vi "EQR reanalysis.vi"() -> ()   [LabVIEW 2015, in "VIPM2.lvlib"]
doc: "El reanàlisi funciona de 2 a 3 condicions, però no al revés; perquè els pixels dolents es sobreescriuen amb els valors de reset del Jose i no són recuperables."
uses:
  VIPM2.lvlib
panel:
  in  "ADC target":u16=900
  in  "TOT":u16=40 caption="us"
  in  "Condition over THLD sweep":bool
  out "summary EQR":string
  out "EQR folder path done":path
  in  "EQ folder path":path
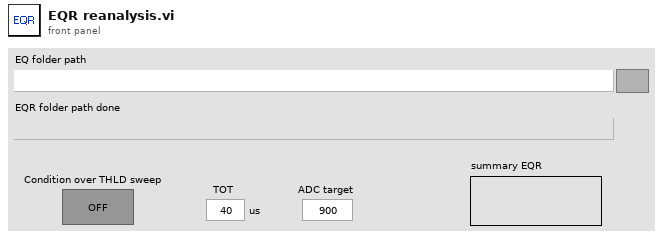
[diagram p1: front panel]
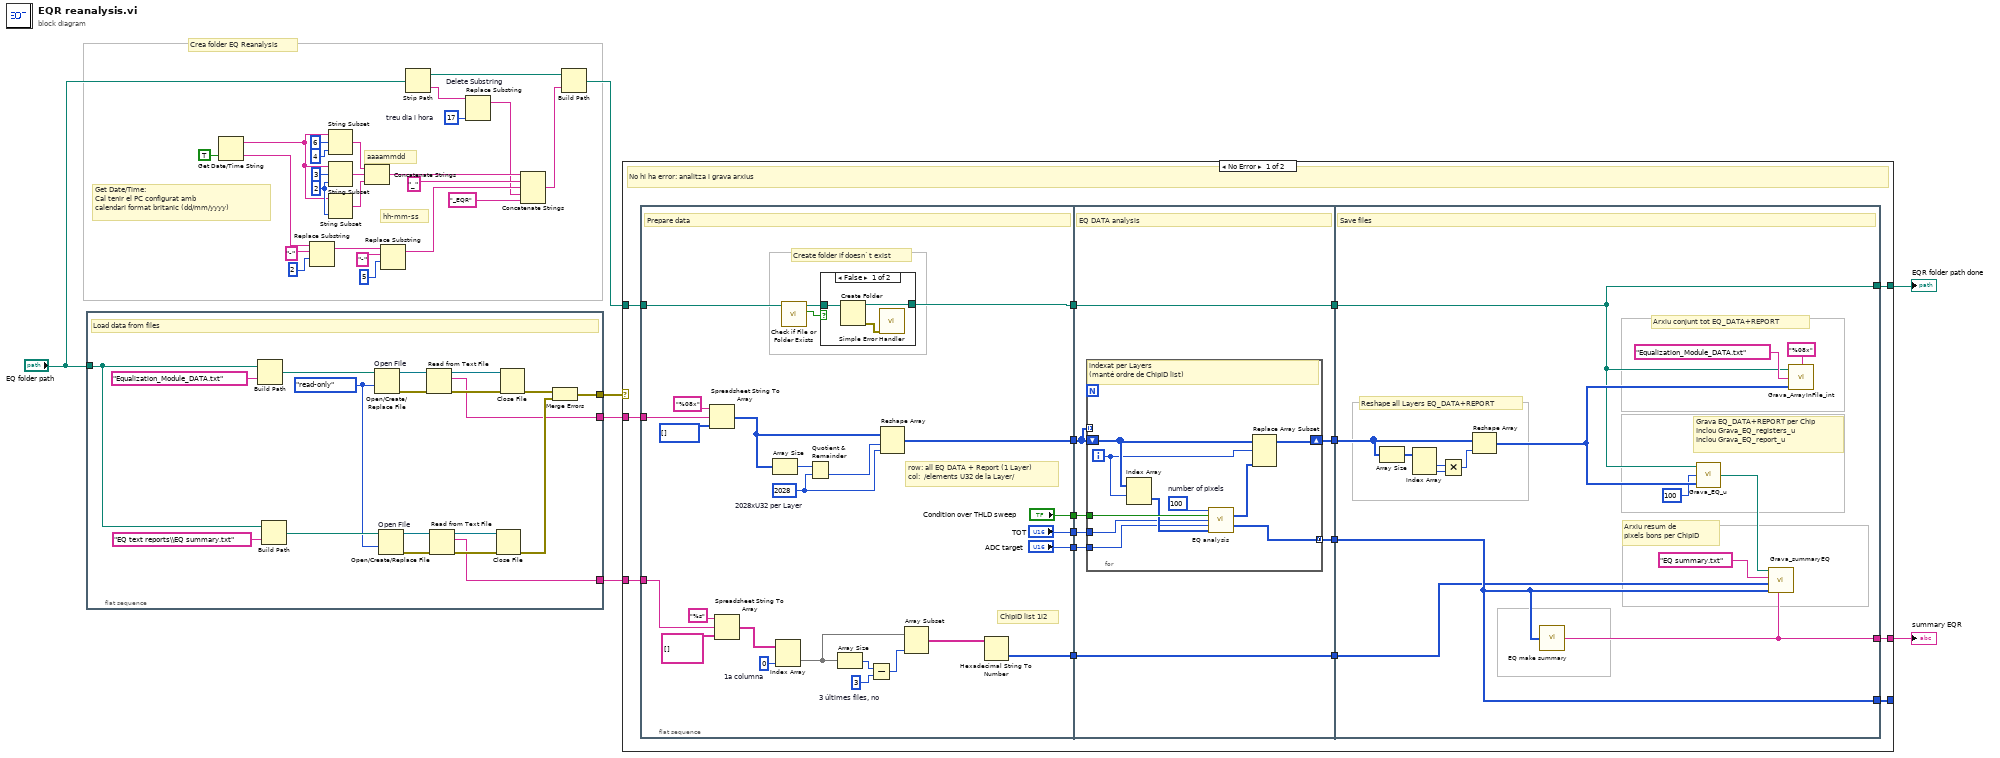
[diagram p0: block diagram]
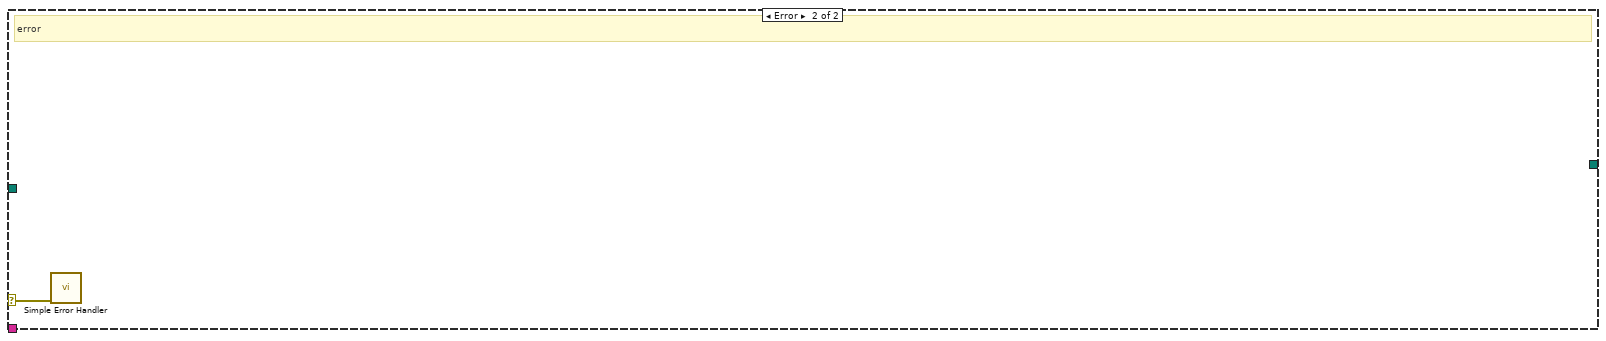
[diagram p3: hidden frame]
diagram:
  w20 = 2 ("length (rest)")
  w27 = 17  # treu dia i hora
  # "Crea folder EQ Reanalysis"
  # "Get Date/Time:\nCal tenir el PC configurat amb\ncalendari format britanic (dd/mm/yyyy)"
  # "hh-mm-ss"
  # "aaaammdd"
  n1 = flat-sequence {
    tunnel: "EQ folder path" -> [w35]
    tunnel: [w45] -> w31
    tunnel: [w33] -> w30
    tunnel: [w32] -> w29
    frame #0 {
      w36 = enum16{"read/write", "read-only", "write-only"}."read-only" ("access (0:read/write)")
      # "Load data from files"
      n2 = Build Path(base path=w35, name or relative path="Equalization_Module_DATA.txt") -> (appended path=w44:path)
      n3 = Build Path(base path=w35, name or relative path="EQ text reports\\EQ summary.txt") -> (appended path=w38:path)
      n4 = Open/Create/Replace File "Open File"(file path (use dialog)=w44, access (0:read/write)=w36) -> (refnum out=w49:refnum<file>, error out=w48:errorcluster)  [unwired: 4 in, 1 out]
      n5 = Open/Create/Replace File "Open File"(file path (use dialog)=w38, access (0:read/write)=w36) -> (refnum out=w39:refnum<file>, error out=w40:errorcluster)  [unwired: 4 in, 1 out]
      n6 = Read from Text File(file (use dialog)=w49, error in=w48) -> (refnum out=w47:refnum<file>, text=w45:string, error out=w46:errorcluster)  [unwired: 2 in, 1 out]
      n7 = Read from Text File(file (use dialog)=w39, error in=w40) -> (refnum out=w41:refnum<file>, text=w32:string, error out=w42:errorcluster)  [unwired: 2 in, 1 out]
      n8 = Close File(refnum=w41, error in=w42) -> (error out=w50:errorcluster)  [unwired: 1 out]
      n9 = Close File(refnum=w47, error in=w46) -> (error out=w34:errorcluster)  [unwired: 1 out]
      n10 = Merge Errors "Merge Errors"(w34, w50) -> (w33:errorcluster)
    }
  }
  n11 = Get Date/Time String(want seconds? (F)=TRUE) -> (date string=w19:string, time string=w24:string)  [unwired: 2 in]
  n12 = Replace Substring(3:2 ("offset (0)"), 4:"-" ("substring (\"\")"), 5:w24) -> (1:w14:string)  [unwired: 1 in, 1 out]
  n13 = String Subset(string=w19, offset (0)=6, length (rest)=4 ("length (rest)")) -> (substring=w21:string)
  n14 = String Subset(string=w19, offset (0)=3, length (rest)=w20) -> (substring=w22:string)
  n15 = String Subset(string=w19, length (rest)=w20) -> (substring=w23:string)  [unwired: 1 in]
  n16 = Concatenate Strings(w21, w22, w23) -> (w11:string)
  n17 = Replace Substring(3:5 ("offset (0)"), 4:"-" ("substring (\"\")"), 5:w14) -> (1:w9:string)  [unwired: 1 in, 1 out]
  n18 = Strip Path(path="EQ folder path") -> (stripped path=w7:path, name=w28:string)
  n19 = Replace Substring "Delete Substring"(2:w27, 5:w28) -> (1:w8:string)  [unwired: 2 in, 1 out]
  n20 = Concatenate Strings "Concatenate Strings"(w11, "_" ("string"), w9, w8, "_EQR" ("string")) -> (w6:string)
  n21 = Build Path(base path=w7, name or relative path=w6) -> (appended path=w3:path)
  n22 = case shown="No Error" w30 {
    selector: w30 -> [_ w130]
    tunnel: [w63 _] -> w2
    tunnel: [w62 _] -> _
    tunnel: [w61 _] -> w1
    tunnel: w31 -> [w60 _]
    tunnel: w29 -> [w59 _]
    tunnel: w3 -> [w55 _]
    frame No Error {
      # "No hi ha error: analitza i grava arxius"
      n23 = flat-sequence {
        tunnel: [w86] -> w66
        tunnel: w60 -> [w85]
        tunnel: w59 -> [w76]
        tunnel: [w74] -> w58
        tunnel: [w70] -> w56
        tunnel: w55 -> [w71]
        tunnel: ["Condition over THLD sweep"] -> w53
        tunnel: ["TOT"] -> w52
        tunnel: ["ADC target"] -> w51
        tunnel: w66 -> [w102]
        tunnel: [w104] -> w65
        tunnel: [w103] -> w64
        tunnel: w58 -> [w101]
        tunnel: [w101] -> w57
        tunnel: w56 -> [w100]
        tunnel: [w100] -> w54
        tunnel: w53 -> [w99]
        tunnel: w52 -> [w98]
        tunnel: w51 -> [w97]
        tunnel: [w115] -> w63
        tunnel: [w119] -> w62
        tunnel: [w118] -> w61
        tunnel: w64 -> [w119]
        tunnel: w65 -> [w125]
        tunnel: w57 -> [w116]
        tunnel: w54 -> [w115]
        frame #0 {
          w84 = 0  # 1a columna
          w79 = 3  # 3 últimes files, no
          w92 = 2028  # 2028xU32 per Layer
          # "Create folder if doesn`t exist"
          # "ChipID list 1i2"
          # "row: all EQ DATA + Report (1 Layer)\ncol:  /elements U32 de la Layer/"
          # "Prepare data"
          n24 = Spreadsheet String To Array(format string="%08x", spreadsheet string=w85, array type (2D Dbl)=u32[] []) -> (array=w89:u32[])  [unwired: 1 in]
          n25 = Spreadsheet String To Array(format string="%s", spreadsheet string=w76, array type (2D Dbl)=string[][] []) -> (array=w81:string[][])  [unwired: 1 in]
          n26 = Array Size(array=w89) -> (size(s)=w90:i32)
          n27 = Index Array "Index Array"(array=w81, index (col)=w84) -> (element=w82:string[])  [unwired: 1 in]
          n28 = call <vilib>:"Check if File or Folder Exists.vi"("path"=w71) -> ("file or folder exists?"=w73:bool, "dup path"=w72:path)  [unwired: 8 in, 1 out]
          n29 = Quotient & Remainder(x=w90, y=w92) -> (floor(x/y)=w91:i32)  [unwired: 1 out]
          n30 = case shown="False" w73 {
            tunnel: w72 -> [w95 w96]
            tunnel: [w94 w96] -> w70
            frame False {
              n31 = Create Folder(path (use dialog)=w95) -> (created path=w94:path, error out=w93:errorcluster)  [unwired: 2 in, 1 out]
              n32 = call <vilib>:"Simple Error Handler.vi"("error in (no error)"=w93) -> ()  [unwired: 4 in, 5 out]
            }
            frame True {
            }
          }
          n33 = Array Size(array=w82) -> (size(s)=w83:i32)
          n34 = Subtract(x=w83, y=w79) -> (x-y=w80:i32)
          n35 = Reshape Array "Reshape Array"(w89, w91, w92) -> (w86:u32[][])
          n36 = Array Subset "Array Subset"(array=w82, length=w80) -> (w75:string[])  [unwired: 1 in]
          n37 = Hexadecimal String To Number(string=w75) -> (number=w74:u32[])  [unwired: 2 in, 1 out]
        }
        frame #1 {
          # "EQ DATA analysis"
          n38 = for {
            shift-right: [w109] -> w104
            shift-left: w102 -> [w111]
            tunnel: [w107] -> w103 mode=concatenating
            tunnel: w102 -> [_] mode=indexing
            tunnel: w99 -> [w114]
            tunnel: w98 -> [w106]
            tunnel: w97 -> [w105]
            i -> [w110]
            w113 = u32 100  # number of pixels
            # "indexat per Layers\n(manté ordre de ChipID list)"
            n39 = Index Array "Index Array"(array=w111, index (row)=w110) -> (element=w112:u32[])  [unwired: 1 in]
            n40 = call "EQ analysis.vi"("number of pixels"=w113, "Condition over THLD sweep"=w114, "TOT (us)"=w106, "ADC target"=w105, "EQ Data and Report"=w112) -> ("EQ Data and Report, analyzed"=w108:u32[], "quants pixels bons per Chip"=w107:u8[])  [unwired: 9 in]
            n41 = Replace Array Subset "Replace Array Subset"(array=w111, new element=w108, index (row)=w110) -> (w109:u32[][])  [unwired: 1 in]
          }
        }
        frame #2 {
          # "Arxiu resum de\npixels bons per ChipID"
          # "Grava EQ_DATA+REPORT per Chip\nInclou Grava_EQ_registers_u\nInclou Grava_EQ_report_u"
          # "Arxiu conjunt tot EQ_DATA+REPORT"
          # "Reshape all Layers EQ_DATA+REPORT"
          # "Save files"
          n42 = Array Size(array=w125) -> (size(s)=w129:i32[])
          n43 = Index Array "Index Array"(array=w129) -> (element #1=w127:i32, element #2=w128:i32)  [unwired: 2 in]
          n44 = Multiply(x=w127, y=w128) -> (x*y=w126:i32)
          n45 = Reshape Array "Reshape Array"(w125, w126) -> (w123:u32[])
          n46 = call "EQ make summary.vi"("quants pixels bons per Chip"=w119) -> ("summary EQ"=w118:string)  [unwired: 4 in]
          n47 = call "Grava_EQ_u.vi"("all Layers EQ_DATA+REPORT"=w123, "number of pixels"=u32 100, "Folder path: equalization"=w115) -> ("subfolder path: text reports"=w121:path)  [unwired: 2 in]
          n48 = call "Grava_summaryEQ.vi"("summary EQ"=w118, "quants pixels bons per Chip"=w119, "ChipID list"=w116, "file name"="EQ summary.txt", "subfolder path: text reports"=w121) -> ()  [unwired: 2 in]
          n49 = call "Grava_ArrayInFile_int.vi"("format (%08x)"="%08x", "Array to save"=w123, "file name"="Equalization_Module_DATA.txt", "folder path"=w115) -> ()  [unwired: 1 in]
        }
      }
    }
    frame Error {
      # "error"
      n50 = call <vilib>:"Simple Error Handler.vi"("error in (no error)"=w130) -> ()  [unwired: 4 in, 5 out]
    }
  }
  "EQR folder path done" <- w2
  "summary EQR" <- w1
